vi "Object Slice.vi"(0 "Image_2d":i16[][](array[numeric]), 2 "Slice Rows(T)/Cols(F)":bool, 5 "error in (no error)":errorcluster, 7 "Threshhold":i32) -> (13 "Object Start/Stop/Sum":i32[](array[numeric]), 14 "Image_2d_Slice":i16[][](array[numeric]), 19 "error out":errorcluster)   [LabVIEW 2016]
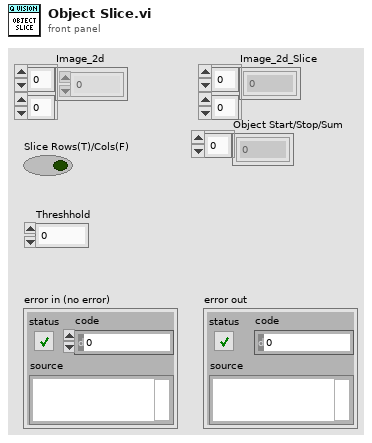
[diagram p1: front panel]
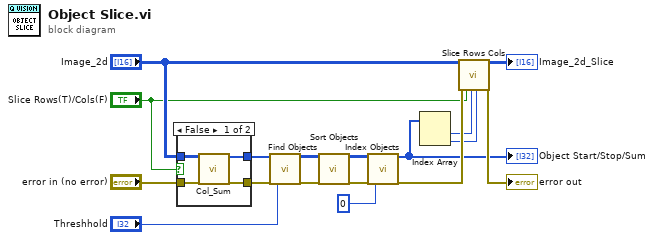
[diagram p0: block diagram]
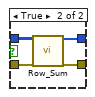
[diagram p2: hidden frame]
diagram:
  n1 = case shown="False" "Slice Rows(T)/Cols(F)" {
    tunnel: "Image_2d" -> [w21 w25]
    tunnel: "error in (no error)" -> [w20 w24]
    tunnel: [w19 w23] -> w8
    tunnel: [w18 w22] -> w7
    frame False {
      n2 = call "Col_Sum.vi"("Image_2d"=w21, "error in (no error)"=w20) -> ("Col_Sum"=w19:i16[], "error out"=w18:errorcluster)  [unwired: 16 in]
    }
    frame True {
      n3 = call "Row_Sum.vi"("Image_2d"=w25, "error in (no error)"=w24) -> ("Row_Sum"=w23:i16[], "error out"=w22:errorcluster)  [unwired: 16 in]
    }
  }
  n4 = call "Find Objects.vi"("RowSum or ColSum"=w8, "error in (no error)"=w7, "Threshhold"="Threshhold") -> ("Object(s) Start/Stop/Sum"=w10:i32[][], "error out"=w9:errorcluster)  [unwired: 15 in]
  n5 = call "Sort Objects.vi"("Object List in"=w10, "error in (no error)"=w9) -> ("Object List out"=w14:i32[][], "error out"=w15:errorcluster)  [unwired: 16 in]
  n6 = call "Index Objects.vi"("Object List in"=w14, "error in (no error)"=w15, "index"=0 ("index (row)")) -> ("Object Start/Stop/Sum"=w3:i32[], "error out"=w6:errorcluster)  [unwired: 15 in]
  "Object Start/Stop/Sum" <- w3
  n7 = Index Array(array=w3) -> (element #1=w2:i32, element #2=w1:i32)  [unwired: 2 in]
  n8 = call "Slice Rows Cols.vi"("Image_2d"="Image_2d", "error in (no error)"=w6, "Slice Rows(T)/Cols(F)"="Slice Rows(T)/Cols(F)", "Start Index"=w2, "Stop Index"=w1) -> ("Image_2d_Slice"=→"Image_2d_Slice":i16[][], "error out"=→"error out":errorcluster)  [unwired: 13 in]
